vi "InitFifo.vi"(8 "error in (no error)":errorcluster, 11 "PmuBase In":refnum<class "PmuBase.lvclass">) -> (0 "error out":errorcluster, 3 "PmuBase Out":refnum<class "PmuBase.lvclass">)   [LabVIEW 2014, in "SensorPlugins.lvlib" / "PmuBase.lvclass"]
uses:
  PmuBase.lvclass
  Typedef/PmuData.ctl
  PmuBase.lvclass/PmuBase.ctl
  Accessors/Read DataFifo.vi
  Accessors/Read PmuConfig.vi
  Accessors/Write DataFifo.vi
  Accessors/Write PmuDataArray.vi
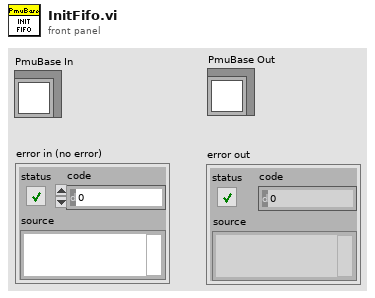
[diagram p1: front panel]
types:
  T1 = typedef "SensorPlugins.lvlib/PmuBase.lvclass/PmuData.ctl" = cluster{"Timestamp":dbl, "Synx":cdb[], "Freq":dbl, "ROCOF":dbl, "ID":i16}
  T2 = typedef "DataFifo.ctl" = cluster{"ReadPointer":u16, "WritePointer":u64, "Locked":bool, "FifoSize":u64}
  T3 = typedef "SensorPlugins.lvlib/PmuBase.lvclass/PmuConfig.ctl" = cluster{"Class":enum16{"M", "P"}, "Fs":i32, "F0":i32, "FSamp":i32, "SettlingTime":dbl, "T0":ext}
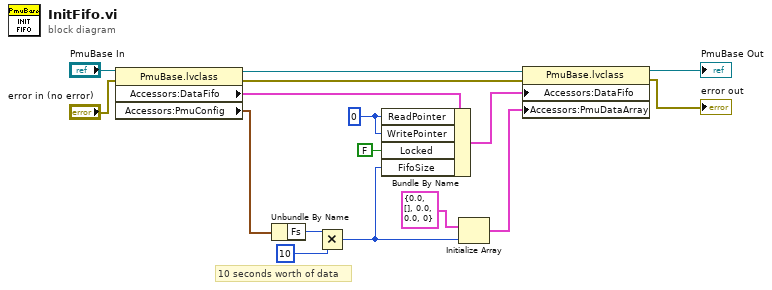
[diagram p0: block diagram]
diagram:
  w6 = u16 0 ("ReadPointer")
  # "10 seconds worth of data"
  n1 = property class="PmuBase.lvclass"(reference="PmuBase In", error in="error in (no error)") -> (reference out=w12:refnum<class "PmuBase.lvclass">, error out=w2:errorcluster, "Accessors:DataFifo"=w9:T2, "Accessors:PmuConfig"=w11:T3)
  n2 = Unbundle By Name(w11) -> ("Fs"=w15:i32)
  n3 = Multiply(x=w15, y=10) -> (x*y=w8:i32)
  n4 = Bundle By Name(cluster=w9, "ReadPointer"=w6, "WritePointer"=w6, "Locked"=FALSE, "FifoSize"=w8) -> (w5:T2)
  n5 = Initialize Array(T1 {"Timestamp"=0.0, "Synx"=[], "Freq"=0.0, "ROCOF"=0.0, "ID"=0} ("PmuReport"), w8) -> (w10:T1[])
  n6 = property class="PmuBase.lvclass"(reference=w12, error in=w2, "Accessors:DataFifo"=w5, "Accessors:PmuDataArray"=w10) -> (reference out=→"PmuBase Out":refnum<class "PmuBase.lvclass">, error out=→"error out":errorcluster)
